vi "VisionDashRead_BackBack.vi"() -> (0 "BB Ang Deg":dbl, 1 "BB Y Ft":dbl, 2 "BB X Ft":dbl, 3 "BB Error":bool, 4 "BB Time Sec":dbl, 5 "BB Conn":bool, 6 "BB Last Sec Cnt":i64, 7 "BB HasTarg":bool, 8 "BB Count":i64, 11 "BB NewData":bool)   [LabVIEW 2023]
doc: "Vision Network\n\nInput\n --Error in \n\nOutput\n --Error out"
uses:
  <vilib>/Rock Robotics/Network Tables/NT Read Integer.vi
  <vilib>/Rock Robotics/Network Tables/NT Read Boolean.vi
  <vilib>/Rock Robotics/Network Tables/NT Read Number.vi
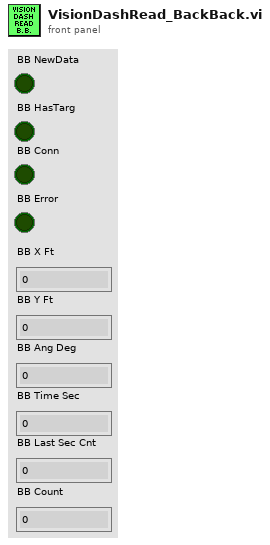
[diagram p1: front panel]
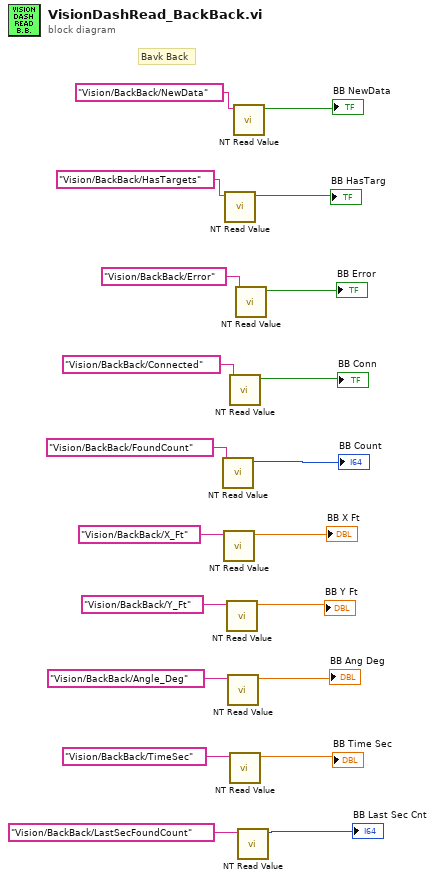
[diagram p0: block diagram]
diagram:
  # "Bavk Back"
  n1 = call-poly <vilib>:"NT Read Value.vi"("name"="Vision/BackBack/FoundCount") -> ("value"=→"BB Count":i64)  [unwired: 8 in, 2 out]
  n2 = call-poly <vilib>:"NT Read Value.vi"("name"="Vision/BackBack/X_Ft") -> ("value"=→"BB X Ft":dbl)  [unwired: 8 in, 2 out]
  n3 = call-poly <vilib>:"NT Read Value.vi"("name"="Vision/BackBack/HasTargets") -> ("value"=→"BB HasTarg":bool)  [unwired: 8 in, 2 out]
  n4 = call-poly <vilib>:"NT Read Value.vi"("name"="Vision/BackBack/Y_Ft") -> ("value"=→"BB Y Ft":dbl)  [unwired: 8 in, 2 out]
  n5 = call-poly <vilib>:"NT Read Value.vi"("name"="Vision/BackBack/Angle_Deg") -> ("value"=→"BB Ang Deg":dbl)  [unwired: 8 in, 2 out]
  n6 = call-poly <vilib>:"NT Read Value.vi"("name"="Vision/BackBack/Connected") -> ("value"=→"BB Conn":bool)  [unwired: 8 in, 2 out]
  n7 = call-poly <vilib>:"NT Read Value.vi"("name"="Vision/BackBack/TimeSec") -> ("value"=→"BB Time Sec":dbl)  [unwired: 8 in, 2 out]
  n8 = call-poly <vilib>:"NT Read Value.vi"("name"="Vision/BackBack/NewData") -> ("value"=→"BB NewData":bool)  [unwired: 8 in, 2 out]
  n9 = call-poly <vilib>:"NT Read Value.vi"("name"="Vision/BackBack/Error") -> ("value"=→"BB Error":bool)  [unwired: 8 in, 2 out]
  n10 = call-poly <vilib>:"NT Read Value.vi"("name"="Vision/BackBack/LastSecFoundCount") -> ("value"=→"BB Last Sec Cnt":i64)  [unwired: 8 in, 2 out]
